vi "oef14.1.vi"() -> ()   [LabVIEW 2021]
uses:
  <vilib>/express/express arith-compare/Formula/XNode/ExpressFormulaBlockNode.xnode
panel:
  out "Waveform Graph":dbl[](graph)
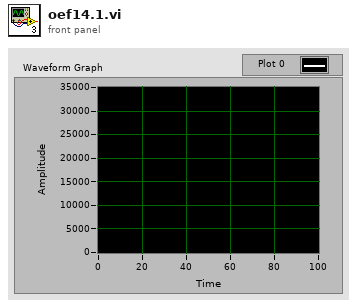
[diagram p1: front panel]
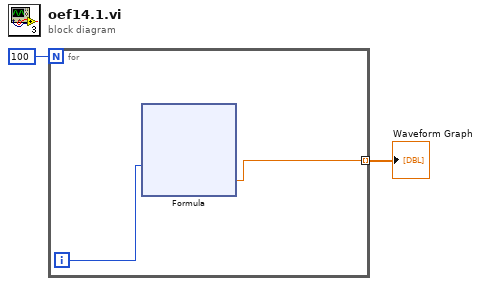
[diagram p0: block diagram]
diagram:
  n1 = for {
    N: 100 -> [_]
    tunnel: [w3] -> w1 mode=indexing
    i -> [w4]
    n2 = xnode "Formula"("X1"=w4) -> ("Result"=w3:dbl)  [unwired: 1 in, 1 out]
  }
  "Waveform Graph" <- w1
